vi "test_ads_surface.vi"() -> ()   [LabVIEW 2017]
doc: "Minimal example that demonstrates functions implemented in the SorpPropLib for adsorption working pairs based on the surface approach."
panel:
  out "Der. of loading wrt. pressure":cluster{dbl[], dbl[]}[](graph)=[{[1000.0, 1001.0, 1002.0, 1003.0, 1004.0, 1005.0, 1006.0, 1007.0, 1008.0, 1009.0], [-1.0, -1.0, -1.0, -1.0, -1.0, -1.0, -1.0, -1.0, -1.0, -1.0]}, {[1000.0, 1001.0, 1002.0, 1003.0, 1004.0, 1005.0, 1006.0, 1007.0, 1008.0, 1009.0], [-1.0, -1.0, -1.0, -1.0, -1.0, -1.0, -1.0, -1.0, -1.0, -1.0]}]
  out "Der. of loading wrt. temperature":cluster{dbl[], dbl[]}[](graph)=[{[1000.0, 1001.0, 1002.0, 1003.0, 1004.0, 1005.0, 1006.0, 1007.0, 1008.0, 1009.0], [-1.0, -1.0, -1.0, -1.0, -1.0, -1.0, -1.0, -1.0, -1.0, -1.0]}, {[1000.0, 1001.0, 1002.0, 1003.0, 1004.0, 1005.0, 1006.0, 1007.0, 1008.0, 1009.0], [-1.0, -1.0, -1.0, -1.0, -1.0, -1.0, -1.0, -1.0, -1.0, -1.0]}]
  out "Der. of pressure wrt. loading":cluster{dbl[], dbl[]}[](graph)=[{[1000.0, 1001.0, 1002.0, 1003.0, 1004.0, 1005.0, 1006.0, 1007.0, 1008.0, 1009.0], [-1.0, -1.0, -1.0, -1.0, -1.0, -1.0, -1.0, -1.0, -1.0, -1.0]}, {[1000.0, 1001.0, 1002.0, 1003.0, 1004.0, 1005.0, 1006.0, 1007.0, 1008.0, 1009.0], [-1.0, -1.0, -1.0, -1.0, -1.0, -1.0, -1.0, -1.0, -1.0, -1.0]}]
  out "Der. of pressure wrt. temperature":cluster{dbl[], dbl[]}[](graph)=[{[1000.0, 1001.0, 1002.0, 1003.0, 1004.0, 1005.0, 1006.0, 1007.0, 1008.0, 1009.0], [-1.0, -1.0, -1.0, -1.0, -1.0, -1.0, -1.0, -1.0, -1.0, -1.0]}, {[1000.0, 1001.0, 1002.0, 1003.0, 1004.0, 1005.0, 1006.0, 1007.0, 1008.0, 1009.0], [-1.0, -1.0, -1.0, -1.0, -1.0, -1.0, -1.0, -1.0, -1.0, -1.0]}]
  out "Temperature":cluster{dbl[], dbl[]}[](graph)=[{[1000.0, 1001.0, 1002.0, 1003.0, 1004.0, 1005.0, 1006.0, 1007.0, 1008.0, 1009.0], [-1.0, -1.0, -1.0, -1.0, -1.0, -1.0, -1.0, -1.0, -1.0, -1.0]}, {[1000.0, 1001.0, 1002.0, 1003.0, 1004.0, 1005.0, 1006.0, 1007.0, 1008.0, 1009.0], [-1.0, -1.0, -1.0, -1.0, -1.0, -1.0, -1.0, -1.0, -1.0, -1.0]}]
  out "Pressure":cluster{dbl[], dbl[]}[](graph)=[{[1000.0, 1001.0, 1002.0, 1003.0, 1004.0, 1005.0, 1006.0, 1007.0, 1008.0, 1009.0], [-1.0, -1.0, -1.0, -1.0, -1.0, -1.0, -1.0, -1.0, -1.0, -1.0]}, {[1000.0, 1001.0, 1002.0, 1003.0, 1004.0, 1005.0, 1006.0, 1007.0, 1008.0, 1009.0], [-1.0, -1.0, -1.0, -1.0, -1.0, -1.0, -1.0, -1.0, -1.0, -1.0]}]
  out "Loading":cluster{dbl[], dbl[]}[](graph)=[{[1000.0, 1001.0, 1002.0, 1003.0, 1004.0, 1005.0, 1006.0, 1007.0, 1008.0, 1009.0], [-1.0, -1.0, -1.0, -1.0, -1.0, -1.0, -1.0, -1.0, -1.0, -1.0]}, {[1000.0, 1001.0, 1002.0, 1003.0, 1004.0, 1005.0, 1006.0, 1007.0, 1008.0, 1009.0], [-1.0, -1.0, -1.0, -1.0, -1.0, -1.0, -1.0, -1.0, -1.0, -1.0]}]
  in  "WorkingPair (Input)":T1={"no_iso"=1, "no_p_sat"=1, "path_db"="D:\\Driesel\\SorpLibLocal\\labview_wrapper\\data\\json\\sorpproplib.json", "wp_as"="zeolite pellet", "wp_st"="5A", "wp_iso"="Toth", "wp_rf"="Water", "rf_rhol"="SaturatedLiquidDensity_EoS1", "no_rhol"=1, "rf_psat"="VaporPressure_EoS1"}
  in  "Temperature in K (Input)":dbl=300.0
  in  "Pressure in Pa (Input)":dbl=1000.0
  # "Increase pressure by 10 Pa in steps of 1 Pa."
  # "Path to database"
  # "Name of sorbent"
  # "Name of sub-type of sorbent"
  # "Name of refrigerant"
  # "Name of isotherm"
  # "ID of isotherm"
  # "Name of calculation approach for vapor pressure"
  # "ID of vapor pressure equation"
  # "Name of calculation approach for liquid density"
  # "ID of liquid density equation"
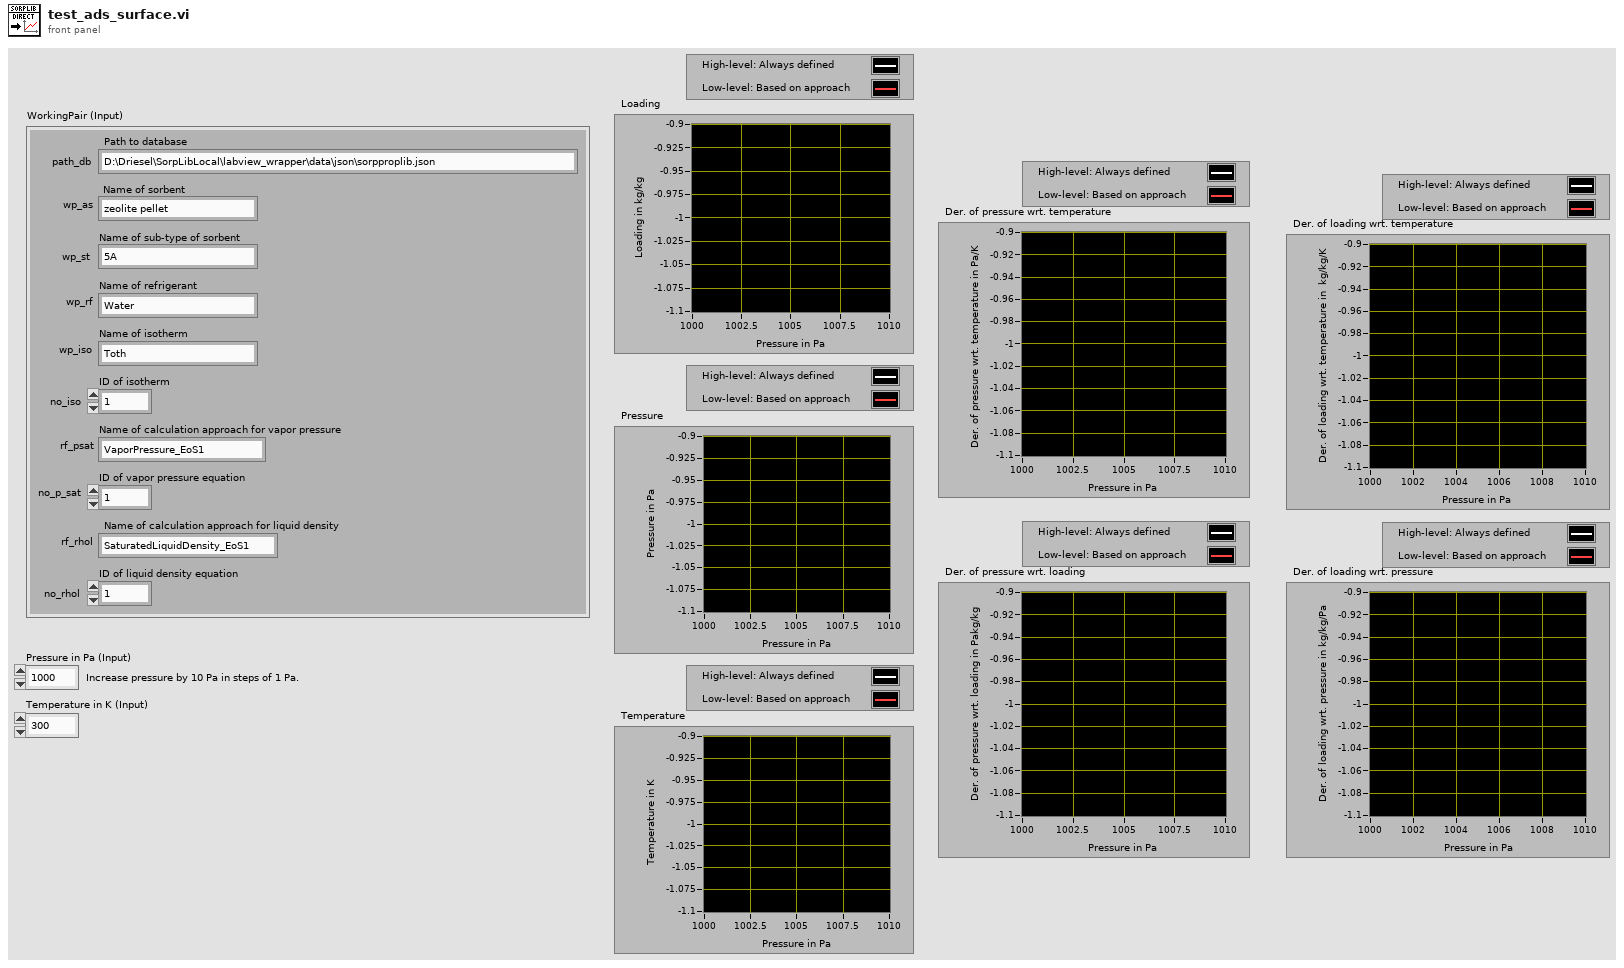
[diagram p1: front panel]
types:
  T1 = cluster{"no_iso":i32, "no_p_sat":i32, "path_db":string, "wp_as":string, "wp_st":string, "wp_iso":string, "wp_rf":string, "rf_rhol":string, "no_rhol":i32, "rf_psat":string}
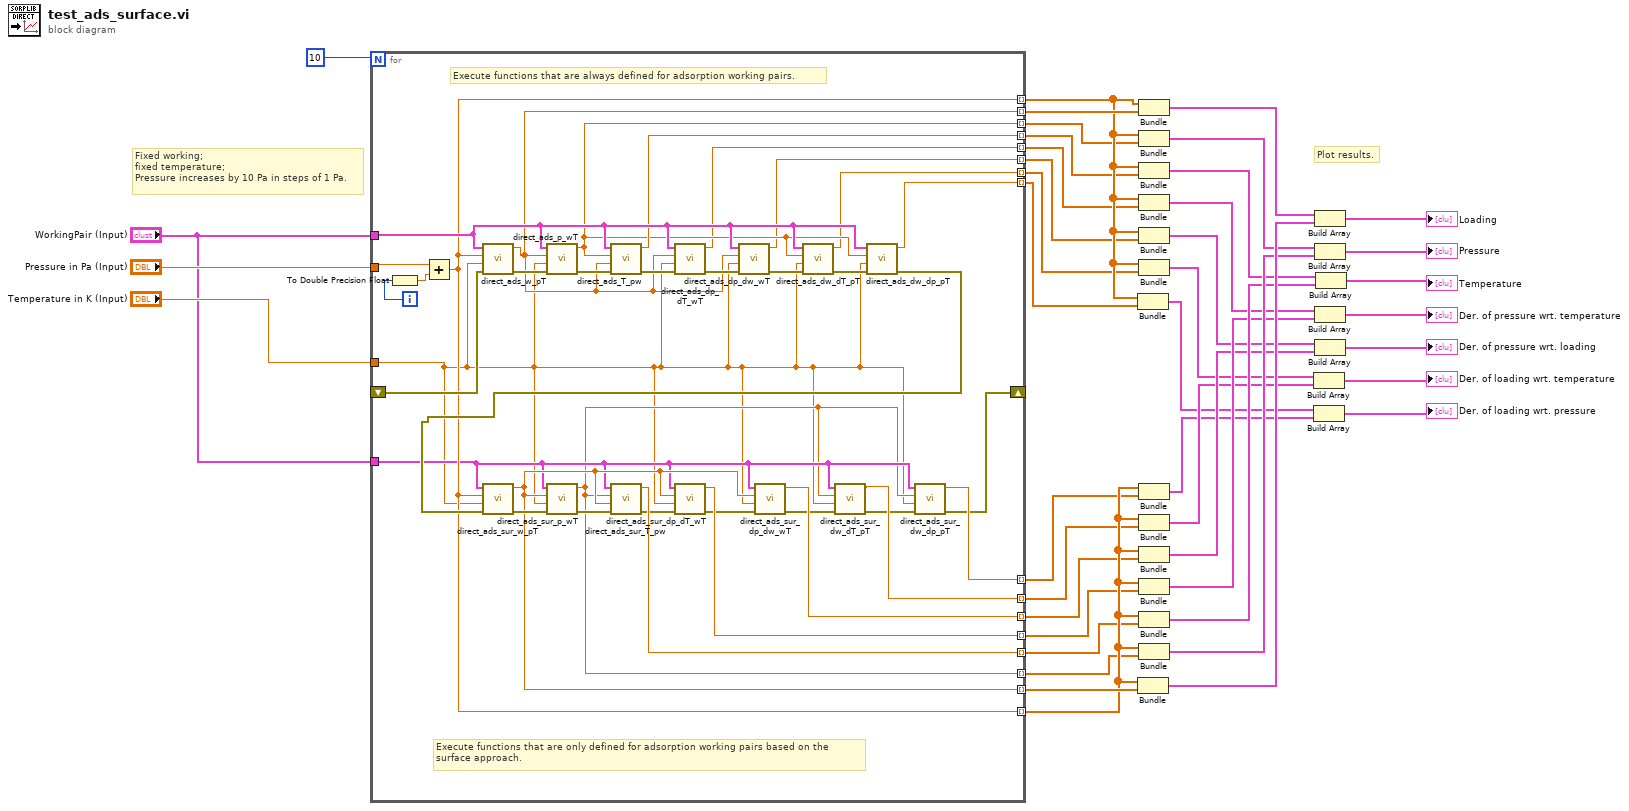
[diagram p0: block diagram]
diagram:
  # "Plot results."
  # "Fixed working;\nfixed temperature;\nPressure increases by 10 Pa in steps of 1 Pa."
  n1 = for {
    N: 10 -> [_]
    tunnel: "Pressure in Pa (Input)" -> [w77]
    tunnel: "Temperature in K (Input)" -> [w43]
    tunnel: "WorkingPair (Input)" -> [w72]
    shift-right: [w42] -> _
    shift-left: _ -> [w60]
    tunnel: [w67] -> w36 mode=indexing
    tunnel: [w58] -> w38 mode=indexing
    tunnel: [w66] -> w39 mode=indexing
    tunnel: [w65] -> w37 mode=indexing
    tunnel: [w64] -> w35 mode=indexing
    tunnel: [w63] -> w34 mode=indexing
    tunnel: [w62] -> w32 mode=indexing
    tunnel: [w61] -> w33 mode=indexing
    tunnel: "WorkingPair (Input)" -> [w46]
    tunnel: [w52] -> w31 mode=indexing
    tunnel: [w58] -> w30 mode=indexing
    tunnel: [w44] -> w29 mode=indexing
    tunnel: [w55] -> w28 mode=indexing
    tunnel: [w53] -> w17 mode=indexing
    tunnel: [w50] -> w14 mode=indexing
    tunnel: [w48] -> w10 mode=indexing
    tunnel: [w45] -> w9 mode=indexing
    i -> [w76]
    # "Execute functions that are only defined for adsorption working pairs based on the\nsurface approach."
    # "Execute functions that are always defined for adsorption working pairs."
    n2 = To Double Precision Float(number=w76) -> (double precision float=w75:dbl)
    n3 = Add(x=w77, y=w75) -> (x+y=w58:dbl)
    n4 = call "direct_ads_w_pT.vi"("Error (Input)"=w60, "Temperature in K (Input)"=w43, "Pressure in Pa (Input)"=w58, "WorkingPair (Input)"=w72) -> ("Error (Output)"=w74:errorcluster, "Loading in kg/kg (Output)"=w66:dbl)  [unwired: 6 in]
    n5 = call "direct_ads_p_wT.vi"("Error (Input)"=w74, "Temperature in K (Input)"=w43, "Loading in kg/kg (Input)"=w66, "WorkingPair (Input)"=w72) -> ("Error (Output)"=w73:errorcluster, "Pressure in Pa (Output)"=w65:dbl)  [unwired: 6 in]
    n6 = call "direct_ads_T_pw.vi"("Error (Input)"=w73, "Loading in kg/kg (Input)"=w66, "Pressure in Pa (Input)"=w65, "WorkingPair (Input)"=w72) -> ("Error (Output)"=w71:errorcluster, "Temperature in K (Output)"=w67:dbl)  [unwired: 6 in]
    n7 = call "direct_ads_dp_dT_wT.vi"("Error (Input)"=w71, "Temperature in K (Input)"=w43, "Loading in kg/kg (Input)"=w66, "WorkingPair (Input)"=w72) -> ("Error (Output)"=w70:errorcluster, "Der. of pressure wrt. temperature in Pa/K (Output)"=w64:dbl)  [unwired: 6 in]
    n8 = call "direct_ads_dp_dw_wT.vi"("Error (Input)"=w70, "Temperature in K (Input)"=w43, "Loading in kg/kg (Input)"=w66, "WorkingPair (Input)"=w72) -> ("Error (Output)"=w69:errorcluster, "Der. of pressure wrt. loading in Pakg/kg (Output)"=w63:dbl)  [unwired: 6 in]
    n9 = call "direct_ads_dw_dT_pT.vi"("Error (Input)"=w69, "Temperature in K (Input)"=w43, "Pressure in Pa (Input)"=w65, "WorkingPair (Input)"=w72) -> ("Error (Output)"=w68:errorcluster, "Der. of loading wrt. temperature in kg/kg/K (Output)"=w62:dbl)  [unwired: 6 in]
    n10 = call "direct_ads_dw_dp_pT.vi"("Error (Input)"=w68, "Temperature in K (Input)"=w43, "Pressure in Pa (Input)"=w65, "WorkingPair (Input)"=w72) -> ("Error (Output)"=w59:errorcluster, "Der. of loading wrt. pressure in kg/kg/Pa (Output)"=w61:dbl)  [unwired: 6 in]
    n11 = call "direct_ads_sur_w_pT.vi"("Error (Input)"=w59, "Temperature in K (Input)"=w43, "Pressure in Pa (Input)"=w58, "WorkingPair (Input)"=w46) -> ("Error (Output)"=w57:errorcluster, "Loading in kg/kg (Output)"=w52:dbl)  [unwired: 6 in]
    n12 = call "direct_ads_sur_p_wT.vi"("Error (Input)"=w57, "Temperature in K (Input)"=w43, "Loading in kg/kg (Input)"=w52, "WorkingPair (Input)"=w46) -> ("Error (Output)"=w56:errorcluster, "Pressure in Pa (Output)"=w44:dbl)  [unwired: 6 in]
    n13 = call "direct_ads_sur_T_pw.vi"("Error (Input)"=w56, "Loading in kg/kg (Input)"=w52, "Pressure in Pa (Input)"=w44, "WorkingPair (Input)"=w46) -> ("Error (Output)"=w54:errorcluster, "Temperature in K (Output)"=w55:dbl)  [unwired: 6 in]
    n14 = call "direct_ads_sur_dp_dT_wT.vi"("Error (Input)"=w54, "Temperature in K (Input)"=w43, "Loading in kg/kg (Input)"=w52, "WorkingPair (Input)"=w46) -> ("Error (Output)"=w51:errorcluster, "Der. pressure wrt. temperature in Pa/K (Output)"=w53:dbl)  [unwired: 6 in]
    n15 = call "direct_ads_sur_dp_dw_wT.vi"("Error (Input)"=w51, "Temperature in K (input)"=w43, "Loading in kg/kg (Input)"=w52, "WorkingPair (Input)"=w46) -> ("Error (Output)"=w49:errorcluster, "Der. pressure wrt. loading in Pakg/kg (Output)"=w50:dbl)  [unwired: 6 in]
    n16 = call "direct_ads_sur_dw_dT_pT.vi"("Error (Input)"=w49, "Temperature in K (input)"=w43, "Pressure in Pa (input)"=w44, "WorkingPair (Input)"=w46) -> ("Error (Output)"=w47:errorcluster, "Der. loading wrt. temperature in kg/kg/K (Output)"=w48:dbl)  [unwired: 6 in]
    n17 = call "direct_ads_sur_dw_dp_pT.vi"("Error (Input)"=w47, "Temperature in K (Input)"=w43, "Pressure in Pa (Input)"=w44, "WorkingPair (Input)"=w46) -> ("Error (Output)"=w42:errorcluster, "Der. loading wrt. pressure in kg/kg/Pa (Output)"=w45:dbl)  [unwired: 6 in]
  }
  n18 = Bundle(w38, w33) -> (w6:cluster{dbl[], dbl[]})  [unwired: 1 in]
  n19 = Bundle(w30, w31) -> (w26:cluster{dbl[], dbl[]})  [unwired: 1 in]
  n20 = Bundle(w38, w39) -> (w27:cluster{dbl[], dbl[]})  [unwired: 1 in]
  n21 = Bundle(w38, w37) -> (w25:cluster{dbl[], dbl[]})  [unwired: 1 in]
  n22 = Bundle(w38, w36) -> (w23:cluster{dbl[], dbl[]})  [unwired: 1 in]
  n23 = Bundle(w38, w35) -> (w21:cluster{dbl[], dbl[]})  [unwired: 1 in]
  n24 = Bundle(w38, w34) -> (w13:cluster{dbl[], dbl[]})  [unwired: 1 in]
  n25 = Bundle(w38, w32) -> (w8:cluster{dbl[], dbl[]})  [unwired: 1 in]
  n26 = Bundle(w30, w9) -> (w5:cluster{dbl[], dbl[]})  [unwired: 1 in]
  n27 = Bundle(w30, w10) -> (w7:cluster{dbl[], dbl[]})  [unwired: 1 in]
  n28 = Bundle(w30, w14) -> (w12:cluster{dbl[], dbl[]})  [unwired: 1 in]
  n29 = Bundle(w30, w17) -> (w16:cluster{dbl[], dbl[]})  [unwired: 1 in]
  n30 = Bundle(w30, w28) -> (w22:cluster{dbl[], dbl[]})  [unwired: 1 in]
  n31 = Bundle(w30, w29) -> (w24:cluster{dbl[], dbl[]})  [unwired: 1 in]
  n32 = Build Array(w8, w7) -> (→"Der. of loading wrt. temperature":cluster{dbl[], dbl[]}[])
  n33 = Build Array(w6, w5) -> (→"Der. of loading wrt. pressure":cluster{dbl[], dbl[]}[])
  n34 = Build Array(w27, w26) -> (→"Loading":cluster{dbl[], dbl[]}[])
  n35 = Build Array(w25, w24) -> (→"Pressure":cluster{dbl[], dbl[]}[])
  n36 = Build Array(w21, w16) -> (→"Der. of pressure wrt. temperature":cluster{dbl[], dbl[]}[])
  n37 = Build Array(w13, w12) -> (→"Der. of pressure wrt. loading":cluster{dbl[], dbl[]}[])
  n38 = Build Array(w23, w22) -> (→"Temperature":cluster{dbl[], dbl[]}[])
